vi "servo_motor_drive_computer.vi"() -> ()   [LabVIEW 2019]
uses:
  <vilib>/Platform/TimedLoop/XDataNode/timing_clust.ctl
  <vilib>/Platform/TimedLoop/XDataNode/nitl_modes.ctl
  <vilib>/Platform/TimedLoop/XDataNode/wakeup.ctl
  <vilib>/Utility/file.llb/Write Delimited Spreadsheet (DBL).vi
  <vilib>/Platform/TimedLoop/XDataNode/XDataNode.xnode
  <vilib>/myRIO/Common/Instrument Driver Framework/Utilities/typedefs/Generic FPGA Reference.ctl
  <vilib>/myRIO/Common/Instrument Driver Framework/Utilities/typedefs/myRIO v1.0 Reference.ctl
  <vilib>/myRIO/Common/Instrument Driver Framework/Utilities/typedefs/Hardware Version Enum.ctl
  <vilib>/myRIO/Common/Instrument Driver Framework/Utilities/typedefs/myRIO Generic Hardware Reference.ctl
  <vilib>/myRIO/Instrument Drivers/Onboard IO/PWM/PWM.lvlib
  <vilib>/myRIO/Instrument Drivers/Onboard IO/PWM/typedefs/PWM Configuration.ctl
  <vilib>/myRIO/Common/Instrument Driver Framework/myRIO v1.0/PWM/typedefs/PWM Channels Enum.ctl
  <vilib>/myRIO/Instrument Drivers/Onboard IO/PWM/typedefs/PWM Reference.ctl
  <vilib>/myRIO/Instrument Drivers/Onboard IO/PWM/vis/myRIO PWM Open.xnode
  <vilib>/myRIO/Instrument Drivers/Utilities/Utilities.lvlib
  <vilib>/myRIO/Common/Instrument Driver Framework/myRIO v1.0/PWM/vis/myRIO v1.1 Open PWM.vi
  <vilib>/userDefined/High Color/nirio_resource_hc.ctl
  <vilib>/myRIO/Express VI/Onboard IO/PWM/PWM Express VI.xnode
  <vilib>/myRIO/Common/Instrument Driver Framework/Utilities/vis/Is FPGA Ref Available.vi
  <vilib>/myRIO/Common/Instrument Driver Framework/myRIO v1.0/Encoder/typedefs/Encoder Count Direction Enum.ctl
  <vilib>/myRIO/Common/Instrument Driver Framework/myRIO v1.0/Encoder/typedefs/Encoder Signal Mode.ctl
  <vilib>/myRIO/Common/Instrument Driver Framework/myRIO v1.0/Encoder/typedefs/Encoder Channels Enum.ctl
  <vilib>/myRIO/Instrument Drivers/Onboard IO/Encoder/typedefs/Encoder Reference.ctl
  <vilib>/myRIO/Instrument Drivers/Onboard IO/Encoder/Encoder.lvlib
  <vilib>/myRIO/Instrument Drivers/Onboard IO/Encoder/vis/Read.vi
  <vilib>/myRIO/Common/Instrument Driver Framework/myRIO v1.0/Encoder/typedefs/Encoder Configuration v1.0.ctl
  <vilib>/myRIO/Common/Instrument Driver Framework/myRIO v1.0/Encoder/vis/myRIO v1.1 Open Encoder.vi
  <vilib>/myRIO/Common/Instrument Driver Framework/myRIO v1.0/Encoder/vis/myRIO v1.0 Configure Encoder.vi
  <vilib>/myRIO/Instrument Drivers/Onboard IO/Encoder/vis/myRIO Encoder Open.xnode
  <vilib>/myRIO/Express VI/Onboard IO/Encoder/Encoder Express VI.xnode
  <vilib>/Platform/TimedLoop/XDataNode/XDNodeRunTimeDep.lvlib
  <vilib>/myRIO/Common/Instrument Driver Framework/myRIO v1.0/DIO/typedefs/DIO Channels Enum.ctl
  <vilib>/myRIO/Common/Instrument Driver Framework/myRIO v1.0/DIO/typedefs/DIO Channels List.ctl
  <vilib>/myRIO/Instrument Drivers/Onboard IO/DIO/typedefs/DIO Reference.ctl
  <vilib>/myRIO/Instrument Drivers/Onboard IO/DIO/DIO.lvlib
  <vilib>/myRIO/Instrument Drivers/Onboard IO/DIO/vis/Write.vi
  <vilib>/myRIO/Common/Instrument Driver Framework/myRIO v1.0/DIO/vis/myRIO v1.1 Open DIO.vi
  <vilib>/myRIO/Instrument Drivers/Onboard IO/DIO/vis/myRIO DIO Open.xnode
  <vilib>/myRIO/Express VI/Onboard IO/DO/DO Express VI.xnode
panel:
  in  "file path (dialog if empty)":path
  in  "format (%.3f)":string="%.3f"
  out "velocity diff (deg/s)":dbl(graph)
  out "angle diff (deg)":dbl(graph)
  out "Duty cycle":dbl(graph)
  out "Time":dbl
  out "Angle_velocity(deg/s)":cluster{"set point":dbl, dbl}(graph)
  out "Angle_velocity(deg/s) Graph":dbl[][](graph)
  out "Angle(deg) Gragh":dbl[][](graph)
  out "Angle(deg)":cluster{dbl, dbl}(graph)
  out "Duty":dbl
  in  "stop":bool
  in  "Frequency [Hz]":dbl=1000.0
  in  "Gain 2":T1={"P Gain"=0.5, "I Gain"=0.0, "D Gain"=0.005}
  out "encoder_position":dbl
  out "Counter Value":i32
  in  "Encoder_Count":dbl=54991.0
  in  "t_shift":dbl=0.000125
  in  "T_ratio":dbl=1.0
  in  "buffer ratio":dbl=0.3
  in  "first or second tripod":bool
  in  "data of 5th order formula\nts,tair,a1-a6":dbl[](array[numeric])
  in  "Loop Period":i64=5
  out "duty cycle[%]":dbl
  out "pulse width[ms]":dbl
  in  "frequency":dbl=100.0
  out "offset":dbl
  in  "null offset":bool
  in  "position":dbl(slide) scale=-30.0..8.0
  in  "PWM channel":tag="A/PWM1"
  in  "stop":bool
  # "RC Servo Motor"
  # "v = 1; a = 15"
  # "v = 1.25; a = 15"
  # "v = 1.5; a = 15"
  # "0.184067181524967\n0.263820978418769\n256152.551336786\n-30272.30000274\n-9876.03760433421\n-1096.38594197941\n885.91817900106\n-44.6781799901984"
  # "0.215241998794118\n0.254514142390288\n4771.41078363533\n62185.8763006578\n-22508.5336527453\n390.805502041188\n686.695311017595\n-40.4128145310291"
  # "0.163616269216122\n0.27489641502463\n771965.39318528\n-201617.027694185\n8828.08396944145\n-2683.04589908678\n1085.57303422127\n-48.5860395324432"
  # "DC Motor"
  # "v = 1.75; a = 15"
  # "v = 2; a = 15"
  # "v = 2.25; a = 15"
  # "0.148651048423414\n0.288542414074344\n1776973.44893281\n-511591.467559457\n38775.9830765103\n-4576.94506688942\n1289.39828252671\n-52.3115561007577"
  # "0.136976185169818\n0.304016701267508\n3461279.85083822\n-993110.73746345\n80544.6579529191\n-6699.48295844177\n1494.82265451498\n-55.8934424469099"
  # "0.134381902205816\n0.369022171779704\n3272804.8365432\n-899365.569589567\n71225.2463409934\n-7039.10791102172\n1512.66147498591\n-59.3408899720725"
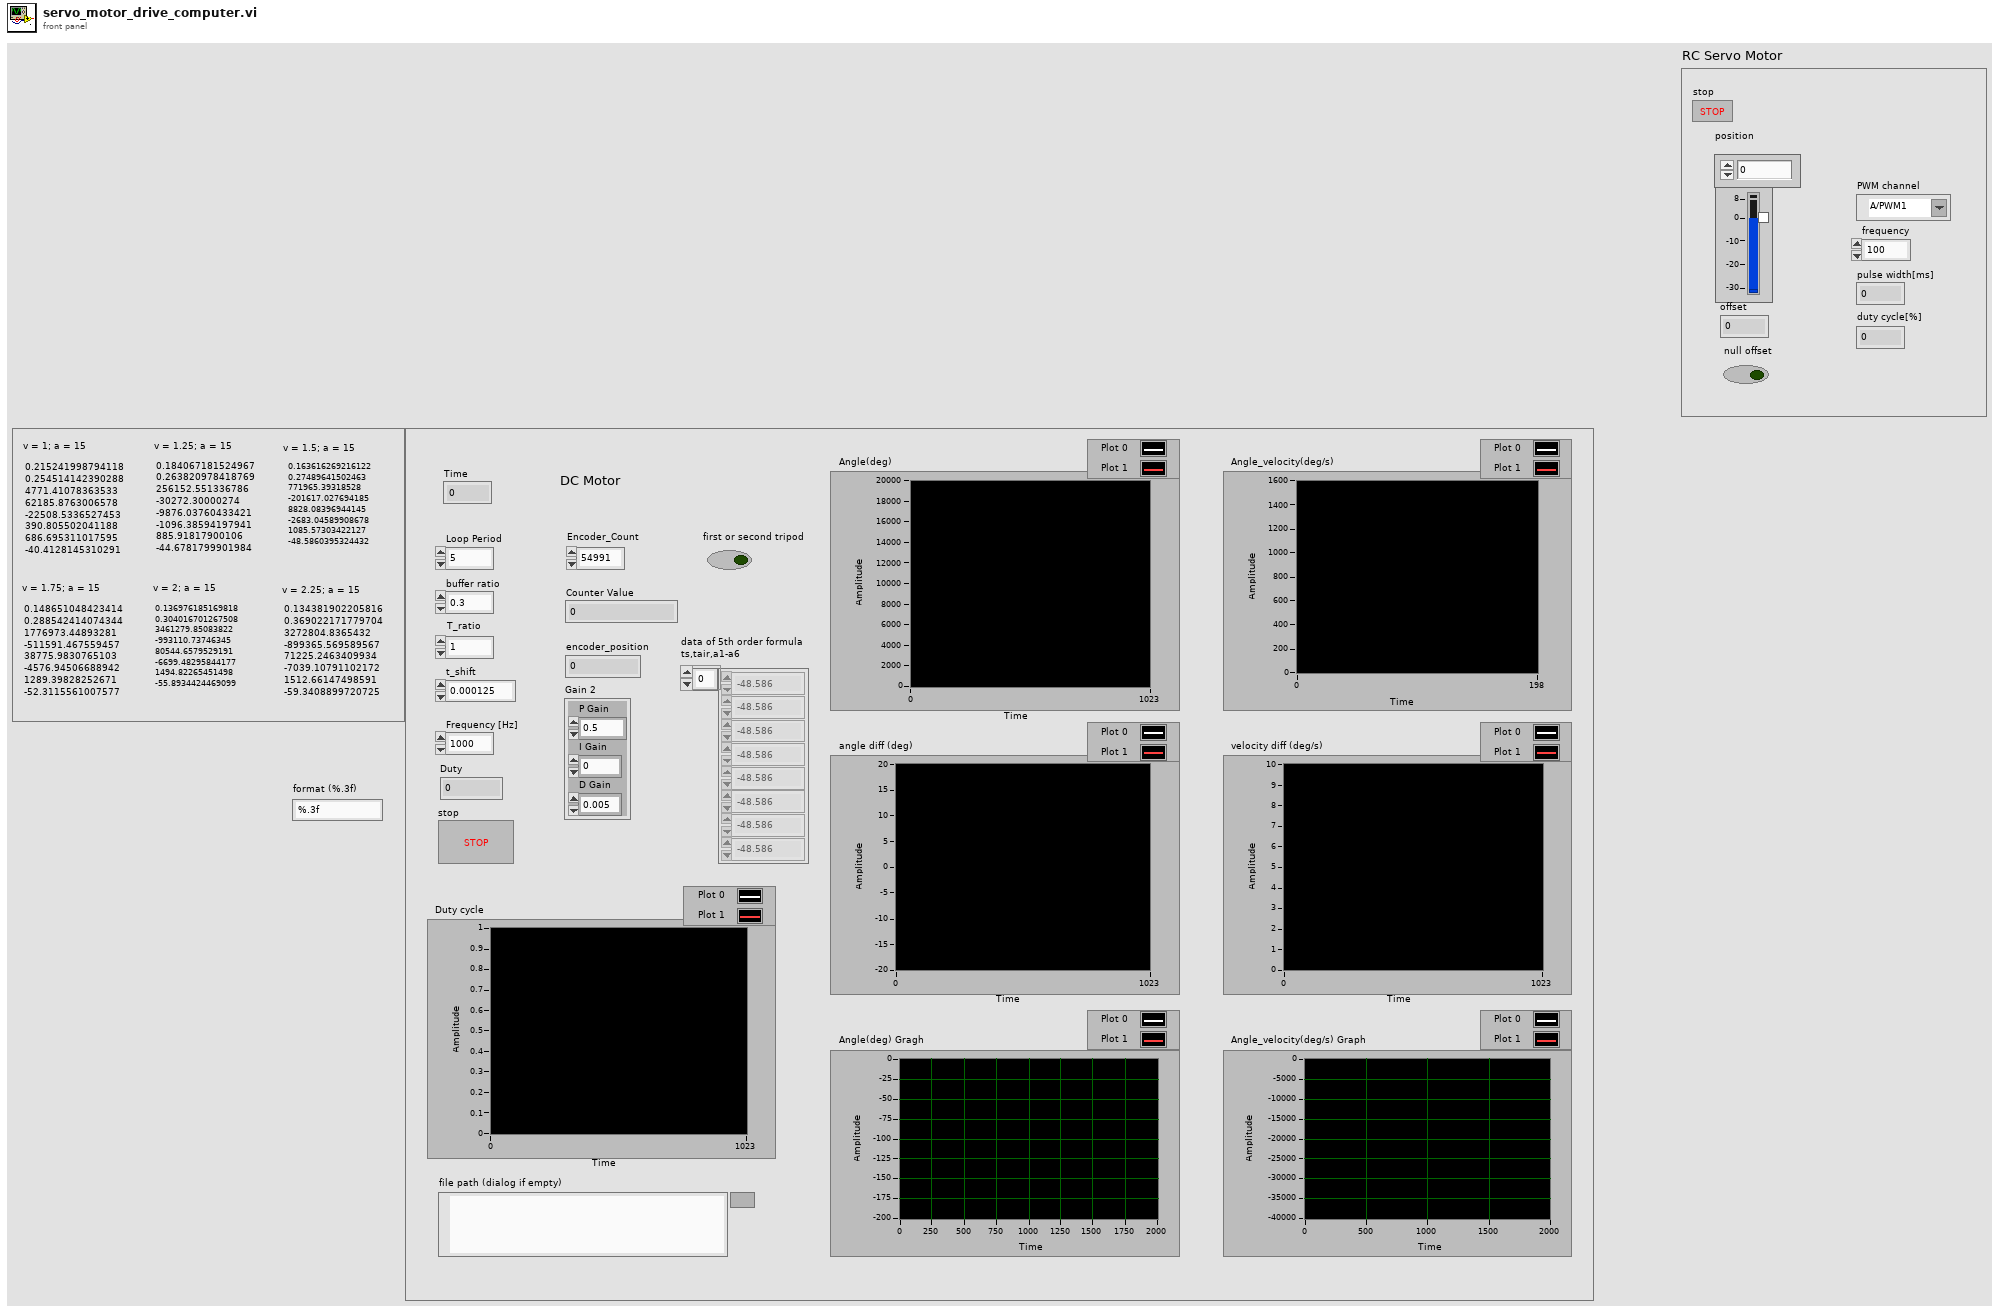
[diagram p1: front panel]
types:
  T1 = cluster{"P Gain":dbl, "I Gain":dbl, "D Gain":dbl}
  T2 = typedef "Encoder.lvlib/Encoder Reference.ctl" = cluster{"myRIO Reference":T3, "Encoder Channels Enum":T7}
  T3 = typedef "myRIO Generic Hardware Reference.ctl" = cluster{"myRIO Model":T4, "myRIO Hardware Reference":T5}
  T4 = typedef "Hardware Version Enum.ctl" = enum16{"Unknown", "myRIO-1900", "myRIO-1950", "roboRIO", "NI ELVIS RIO CM", "ELVIS III"}
  T5 = typedef "myRIO v1.0 Reference.ctl" = cluster{"Generic FPGA Reference":T6, "Allow multiple opens":bool}
  T6 = typedef "Generic FPGA Reference.ctl" = refnum<k20>
  T7 = typedef "Encoder Channels Enum.ctl" = enum16{"Not Connected", "C/ENC0", "C/ENC1", "A/ENC", "A/ENC0", "A/ENC1", "A/ENC2", "A/ENC3", "A/ENC4", "A/ENC5", "A/ENC6", "A/ENC7", "A/ENC8", "A/ENC9", "B/ENC", "B/ENC0", "B/ENC1", "B/ENC2", "B/ENC3", "B/ENC4", "B/ENC5", "B/ENC6", "B/ENC7", "B/ENC8", "B/ENC9", "DIO/ENC0", "DIO/ENC1", "DIO/ENC2", "DIO/ENC3", "DIO/ENC4"}
  T8 = typedef "Encoder Signal Mode.ctl" = enum16{"Quadrature phase signal", "Step and direction signal"}
  T9 = typedef "nirio_resource_hc.ctl" = tag
  T10 = cluster{"set position":dbl, "set position":dbl, "set position":dbl, "set position":dbl, "set position":dbl, "set position":dbl}
  T11 = typedef "PWM.lvlib/PWM Reference.ctl" = cluster{"myRIO Reference":T3, "PWM Channels Enum":T12, "PWM Configuration":T13}
  T12 = typedef "PWM Channels Enum.ctl" = enum16{"Not Connected", "C/PWM0", "C/PWM1", "A/PWM0", "A/PWM1", "A/PWM2", "A/PWM3", "A/PWM4", "A/PWM5", "A/PWM6", "A/PWM7", "A/PWM8", "A/PWM9", "A/PWM10", "A/PWM11", "A/PWM12", "A/PWM13", "A/PWM14", "A/PWM15", "A/PWM16", "A/PWM17", "A/PWM18", "A/PWM19", "B/PWM0", "B/PWM1", "B/PWM2", "B/PWM3", "B/PWM4", "B/PWM5", "B/PWM6", "B/PWM7", "B/PWM8", "B/PWM9", "B/PWM10", "B/PWM11", "B/PWM12", "B/PWM13", "B/PWM14", "B/PWM15", "B/PWM16", "B/PWM17", "B/PWM18", "B/PWM19", "PWM/PWM0", "PWM/PWM1", "PWM/PWM2", "PWM/PWM3", "PWM/PWM4", "PWM/PWM5", "PWM/PWM6", "PWM/PWM7", "PWM/PWM8", "PWM/PWM9"}
  T13 = typedef "PWM.lvlib/PWM Configuration.ctl" = cluster{"Frequency":dbl, "Duty Cycle":dbl}
  T14 = typedef "DIO.lvlib/DIO Reference.ctl" = cluster{"myRIO Reference":T3, "DIO Channels List":T15}
  T15 = typedef "DIO Channels List.ctl" = T16[]
  T16 = typedef "DIO Channels Enum.ctl" = enum16{"Not Connected", "C/DIO0", "C/DIO1", "C/DIO2", "C/DIO3", "C/DIO4", "C/DIO5", "C/DIO6", "C/DIO7", "A/DIO0", "A/DIO1", "A/DIO2", "A/DIO3", "A/DIO4", "A/DIO5", "A/DIO6", "A/DIO7", "A/DIO8", "A/DIO9", "A/DIO10", "A/DIO11", "A/DIO12", "A/DIO13", "A/DIO14", "A/DIO15", "A/DIO16", "A/DIO17", "A/DIO18", "A/DIO19", "B/DIO0", "B/DIO1", "B/DIO2", "B/DIO3", "B/DIO4", "B/DIO5", "B/DIO6", "B/DIO7", "B/DIO8", "B/DIO9", "B/DIO10", "B/DIO11", "B/DIO12", "B/DIO13", "B/DIO14", "B/DIO15", "B/DIO16", "B/DIO17", "B/DIO18", "B/DIO19", "LED0", "LED1", "LED2", "LED3", "Button0", "DIO/DIO0", "DIO/DIO1", "DIO/DIO2", "DIO/DIO3", "DIO/DIO4", "DIO/DIO5", "DIO/DIO6", "DIO/DIO7", "DIO/DIO8", "DIO/DIO9", "SPI/CS0", "SPI/CS1", "SPI/CS2", "SPI/CS3", "LED RADIO (Green)", "LED RADIO (Red)", "LED COMM (Green)", "LED COMM (Red)", "LED MODE (Green)", "LED MODE (Red)"}
  T17 = typedef "XDNodeRunTimeDep.lvlib/timing_clust.ctl" = cluster{"Expected End [f-1]":u64, "Actual End [f-1]":u64, "Finished Late? [f-1]":bool, "Expected End [i-1]":u64, "Actual End [i-1]":u64, "Finished Late? [i-1]":bool, "Expected Start [i]":u64, "Actual Start [i]":u64, "Expected Start [f]":u64, "Actual Start [f]":u64, "Source Name":string, "Structure Name":string, "Period":i64, "Deadline":i64, "Offset":i64, "Start":i64, "Priority":i32, "Timeout":i32, "Mode":T18, "Wakeup Reason":T19, "Error":errorcluster, "Source Type":string, "Secondary Source Type":string, "Global End Time":u64, "Global Start Time":u64, "Frame Duration":u64, "Iteration Duration":u64, "Assigned CPU":i32, "I/O Scan Engine Mode":u32}
  T18 = typedef "XDNodeRunTimeDep.lvlib/nitl_modes.ctl" = enum32{"No Change", "Process missed periods, maintain original phase", "Discard missed periods, maintain original phase", "Process missed periods, ignore original phase", "Discard missed periods, ignore original phase"}
  T19 = typedef "XDNodeRunTimeDep.lvlib/wakeup.ctl" = enum32{"Normal", "Aborted", "Asynchronous wakeup", "Timing source error", "Timed loop error", "Timeout"}
  T20 = cluster{"[0]":dbl, "[1]":dbl, "[2]":dbl, "[3]":dbl, "[4]":dbl, "[5]":dbl}
  T21 = cluster{"set position":i32, "set position":i32, "set position":i32, "set position":i32, "set position":i32, "set position":i32}
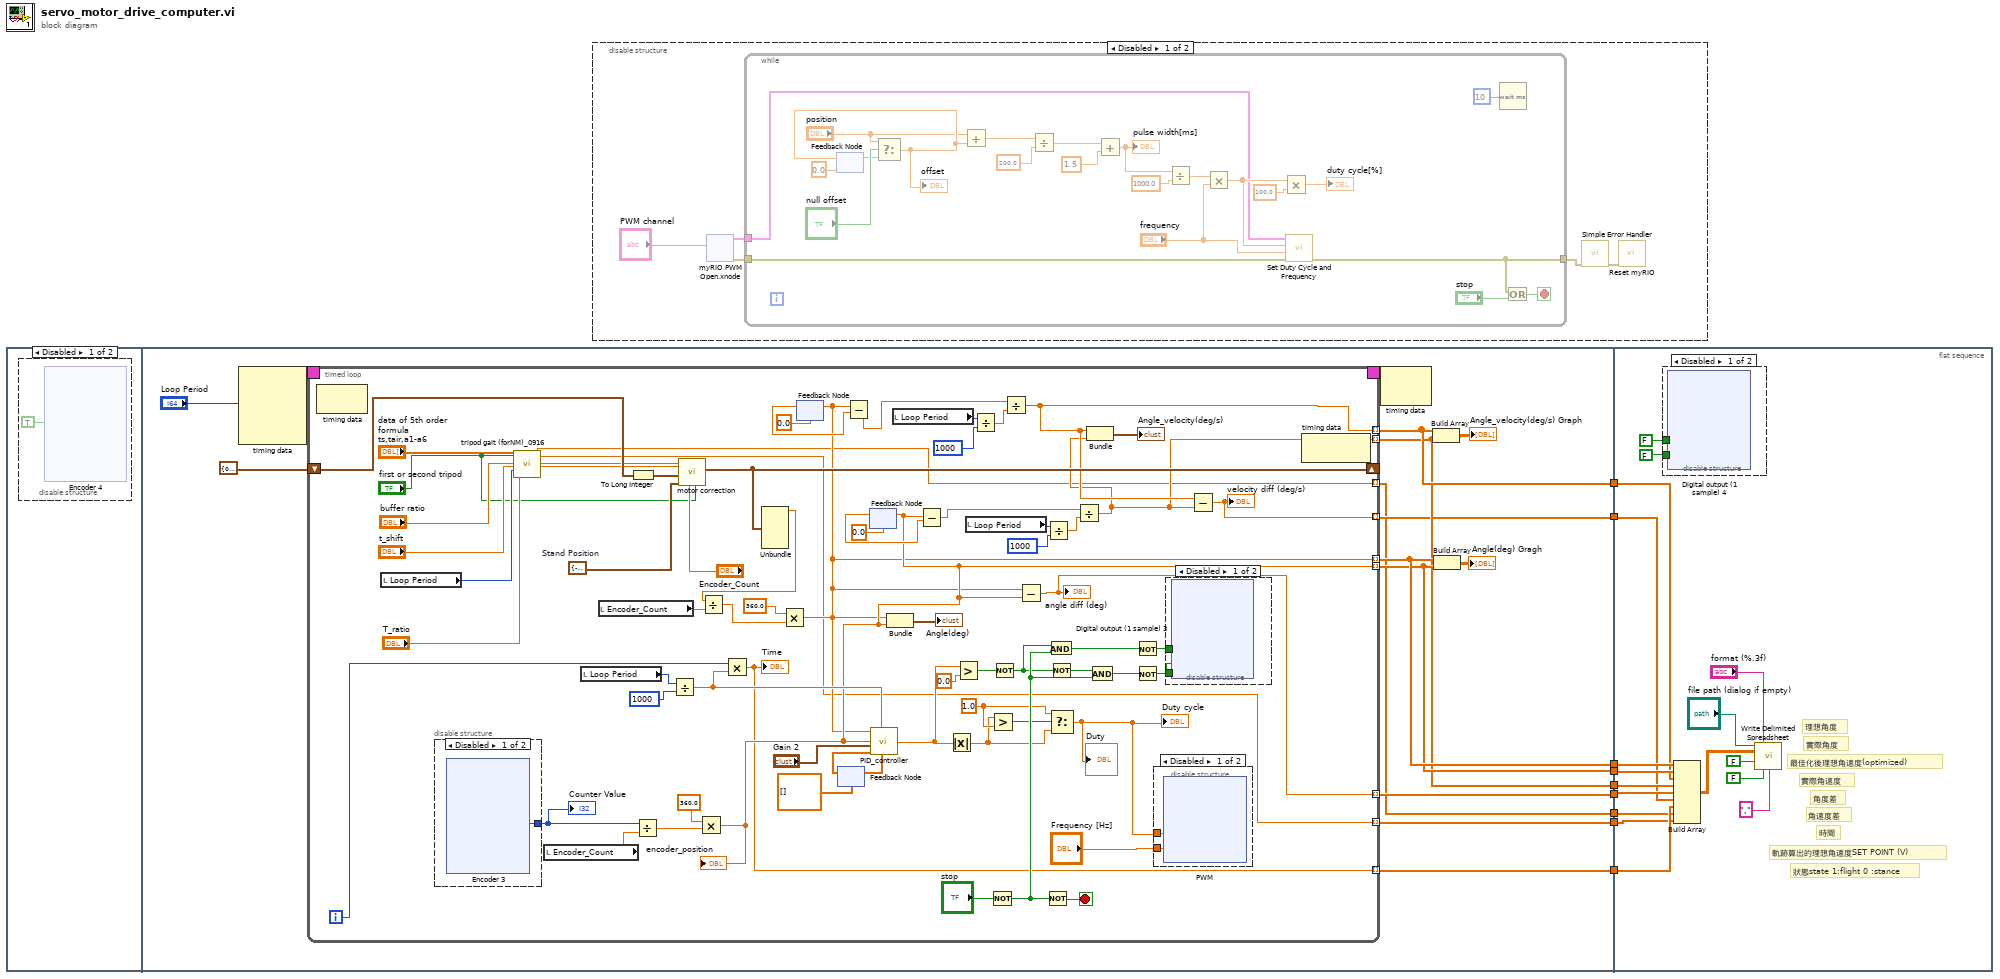
[diagram p0: block diagram]
diagram:
  n1 = flat-sequence {
    tunnel: [w65] -> w9
    tunnel: [w64] -> w8
    tunnel: [w63] -> w7
    tunnel: [w62] -> w6
    tunnel: [w61] -> w5
    tunnel: [w60] -> w4
    tunnel: [w59] -> w3
    tunnel: [w58] -> w2
    tunnel: [w57] -> w1
    tunnel: w9 -> [w282]
    tunnel: w8 -> [w281]
    tunnel: w7 -> [w280]
    tunnel: w6 -> [w279]
    tunnel: w5 -> [w278]
    tunnel: w4 -> [w277]
    tunnel: w3 -> [w275]
    tunnel: w2 -> [w270]
    tunnel: w1 -> [w269]
    frame #0 {
      n2 = disable-structure shown="Disabled" {
        frame Disabled {
          n3 = xnode "Encoder 4"("Reset Counter"=TRUE) -> ()  [unwired: 1 in, 4 out]
        }
        frame Enabled {
        }
      }
    }
    frame #1 {
      n4 = node-c288("Loop Period") -> (w71:T17)  [unwired: 3 in]
      n5 = timed-loop {
        timing: w71 -> [_]
        timing-out: [_] -> w70
        shift-right: [w132] -> _
        shift-left: T10 {"set position"=0.0, "set position"=0.0, "set position"=0.0, "set position"=0.0, "set position"=0.0, "set position"=0.0} ("Setpoint_to_motor") -> [w130]
        tunnel: [w82] -> w64 mode=indexing
        tunnel: [w79] -> w65 mode=indexing
        tunnel: [w80] -> w62 mode=indexing
        tunnel: [w81] -> w63 mode=indexing
        tunnel: [w78] -> w61 mode=indexing
        tunnel: [w77] -> w60 mode=indexing
        tunnel: [w76] -> w59 mode=indexing
        tunnel: [w75] -> w58 mode=indexing
        tunnel: [w74] -> w57 mode=indexing
        i -> [w89]
        stop <- w109 stop-if-true
        w117 = 1.0 ("y")
        w129 = T20 {"[0]"=-27495.5, "[1]"=-27495.5, "[2]"=-27495.5, "[3]"=-27495.5, "[4]"=-27495.5, "[5]"=-27495.5}  # Stand Position
        n6 = node-c288() -> ()  [unwired: 1 in, 1 out]
        n7 = local read "Loop Period"() -> (w136:i64)
        n8 = disable-structure shown="Disabled" {
          disable-tunnel: [w216 _] -> w84
          frame Disabled {
            n9 = xnode "Encoder 3"() -> ("Counter Value"=w216:i32)  [unwired: 2 in, 3 out]
          }
          frame Enabled {
          }
        }
        "Counter Value" <- w84
        n10 = call "tripod gait (forNM)_0916.vi"("data of 5th order formula\nts,tair,a1-a6"="data of 5th order formula\nts,tair,a1-a6", "first or second"="first or second tripod", "buffer ratio"="buffer ratio", "t_shift"="t_shift", "sample time"=w136, "T_ratio"="T_ratio") -> ("SET POINT V"=w75:dbl, "state 2"=w74:dbl, "Set Point"=w73:dbl, "Set Point 2"=w92:dbl)  [unwired: 4 in, 14 out]
        n11 = local read "Encoder_Count"() -> (w133:dbl)
        n12 = local read "Loop Period"() -> (w100:i64)
        n13 = local read "Encoder_Count"() -> (w98:dbl)
        n14 = To Long Integer(number=w130) -> (32bit integer=w131:T21)
        n15 = Divide(x=w84, y=w133) -> (x/y=w93:dbl)
        n16 = Divide(x=w100, y=i64 1000) -> (x/y=w90:dbl)
        n17 = call "motor correction.vi"("first or second"="first or second tripod", "Encoder_Count"="Encoder_Count", "Stand Position"=w129, "encoder position"=w131, "set position 2"=w92, "set position"=w73) -> ("Setpoint_to_motor"=w132:T10)  [unwired: 4 in, 1 out]
        n18 = Multiply(x=360.0, y=w93) -> (x*y=w82:dbl)
        "encoder_position" <- w82
        n19 = Multiply(x=w89, y=w90) -> (x*y=w76:dbl)
        "Time" <- w76
        n20 = Unbundle(w132) -> ("set position"=w72:dbl)  [unwired: 5 out]
        n21 = Divide(x=w72, y=w98) -> (x/y=w96:dbl)
        n22 = Multiply(x=360.0, y=w96) -> (x*y=w79:dbl)
        n23 = feedback #1(0.0) -> (w104:dbl)
        n24 = feedback-in #1(w79) -> ()
        n25 = feedback #2(dbl[] [] ("state(k)")) -> (w128:dbl[])
        n26 = Subtract(x=w79, y=w104) -> (x-y=w87:dbl)
        n27 = feedback #3(0.0) -> (w86:dbl)
        n28 = feedback-in #3(w82) -> ()
        n29 = call "PID_controller.vi"("Time Period"=w90, "state(k-1)"=w128, "Gain"="Gain 2", "variable"=w82, "set point"=w79) -> ("PID gain"=w110:dbl, "state(k)"=w127:dbl[])
        n30 = feedback-in #2(w127) -> ()
        n31 = Bundle(w79, w82) -> (→"Angle(deg)":cluster{dbl, dbl})  [unwired: 1 in]
        n32 = local read "Loop Period"() -> (w103:i64)
        n33 = Subtract(x=w82, y=w86) -> (x-y=w88:dbl)
        n34 = Absolute Value(x=w110) -> (abs(x)=w116:dbl)
        n35 = Greater?(x=w110, y=0.0) -> (0:w119:bool)
        n36 = local read "Loop Period"() -> (w107:i64)
        n37 = Divide(x=w103, y=i64 1000) -> (x/y=w102:dbl)
        n38 = Not(x="stop") -> (.not. x?=w121:bool)
        n39 = Greater?(x=w116, y=w117) -> (0:w118:bool)
        n40 = Not(x=w119) -> (.not. x?=w115:bool)
        n41 = Divide(x=w87, y=w102) -> (x/y=w81:dbl)
        n42 = Subtract(x=w79, y=w82) -> (x-y=w78:dbl)
        "angle diff (deg)" <- w78
        n43 = Not(x=w121) -> (.not. x?=w109:bool)
        n44 = Divide(x=w107, y=i64 1000) -> (x/y=w105:dbl)
        n45 = And(x=w115, y=w121) -> (x .and. y?=w112:bool)
        n46 = Not(x=w115) -> (.not. x?=w123:bool)
        n47 = Select(t=w117, s=w118, f=w116) -> (s? t:f=w83:dbl)
        "Duty" <- w83
        "Duty cycle" <- w83
        n48 = Divide(x=w88, y=w105) -> (x/y=w80:dbl)
        n49 = Bundle(w81, w80) -> (→"Angle_velocity(deg/s)":cluster{dbl, dbl})  [unwired: 1 in]
        n50 = And(x=w123, y=w121) -> (x .and. y?=w114:bool)
        n51 = Not(x=w112) -> (.not. x?=w111:bool)
        n52 = Not(x=w114) -> (.not. x?=w113:bool)
        n53 = disable-structure shown="Disabled" {
          disable-tunnel: "Frequency [Hz]" -> [w142 _]
          disable-tunnel: w83 -> [w141 _]
          frame Disabled {
            n54 = xnode "PWM"("Duty Cycle"=w141, "Frequency [Hz]"=w142) -> ()  [unwired: 1 in, 1 out]
          }
          frame Enabled {
          }
        }
        n55 = disable-structure shown="Disabled" {
          disable-tunnel: w113 -> [w179 _]
          disable-tunnel: w111 -> [w178 _]
          frame Disabled {
            n56 = xnode "Digital output (1 sample) 3"("A/DIO0 (Pin 11)"=w178, "A/DIO1 (Pin 13)"=w179) -> ()  [unwired: 1 in, 1 out]
          }
          frame Enabled {
          }
        }
        n57 = Subtract(x=w81, y=w80) -> (x-y=w77:dbl)
        "velocity diff (deg/s)" <- w77
        n58 = node-c288() -> ()  [unwired: 1 in, 1 out]
      }
      n59 = node-c288(w70) -> ()  [unwired: 1 out]
      n60 = Build Array(w63, w62) -> (→"Angle_velocity(deg/s) Graph":dbl[][])
      n61 = Build Array(w65, w64) -> (→"Angle(deg) Gragh":dbl[][])
    }
    frame #2 {
      # "狀態state 1:flight 0 :stance"
      # "軌跡算出的理想角速度SET POINT (V)"
      # "時間"
      # "角速度差"
      # "角度差"
      # "實際角度"
      # "理想角度"
      # "實際角速度"
      # "最佳化後理想角速度(optimized)"
      n62 = disable-structure shown="Disabled" {
        disable-tunnel: FALSE ("A/DIO0 (Pin 11)") -> [w287 _]
        disable-tunnel: FALSE ("A/DIO1 (Pin 13)") -> [w286 _]
        frame Disabled {
          n63 = xnode "Digital output (1 sample) 4"("A/DIO0 (Pin 11)"=w287, "A/DIO1 (Pin 13)"=w286) -> ()  [unwired: 1 in, 1 out]
        }
        frame Enabled {
        }
      }
      n64 = Build Array(w282, w281, w280, w279, w278, w277, w275, w270, w269) -> (w276:dbl[][])
      n65 = call-poly <vilib>:"Write Delimited Spreadsheet.vi"("file path (dialog if empty)"="file path (dialog if empty)", "format (%.3f)"="format (%.3f)", "2D data"=w276, "append to file? (new file:F)"=FALSE, "transpose? (no:F)"=FALSE, "delimiter (\\t)"="," ("delimiter (\\t)")) -> ()  [unwired: 8 in, 2 out]
    }
  }
  n66 = disable-structure shown="Disabled" {
    frame Disabled {
      n67 = xnode "myRIO PWM Open.xnode"("Channel Name"="PWM channel") -> ("error out"=w326:errorcluster, "PWM Ref Out"=w327:T11)  [unwired: 2 in]
      n68 = while {
        tunnel: w327 -> [w351]
        tunnel: w326 -> [w350]
        tunnel: [w349] -> w325
        stop <- w347 stop-if-true
        n69 = feedback #4(0.0 ("Numeric")) -> (w364:dbl)
        n70 = Select(t="position", s="null offset", f=w364) -> (s? t:f=w363:dbl)
        "offset" <- w363
        n71 = feedback-in #4(w363) -> ()
        n72 = Add(x="position", y=w363) -> (x+y=w362:dbl)
        n73 = Divide(x=w362, y=200.0) -> (x/y=w360:dbl)
        n74 = Add(x=w360, y=1.5) -> (x+y=w358:dbl)
        "pulse width[ms]" <- w358
        n75 = Divide(x=w358, y=1000.0) -> (x/y=w356:dbl)
        n76 = Multiply(x=w356, y="frequency") -> (x*y=w354:dbl)
        n77 = Multiply(x=w354, y=100.0) -> (x*y=→"duty cycle[%]":dbl)
        n78 = call <vilib>:"Set Duty Cycle and Frequency.vi"("error in (no error)"=w350, "Frequency [Hz]"="frequency", "Duty Cycle"=w354, "PWM Ref In"=w351) -> ("error out"=w349:errorcluster)  [unwired: 5 in, 1 out]
        n79 = Wait (ms)(milliseconds to wait=u32 10) -> ()  [unwired: 1 out]
        n80 = Or(x=w349, y="stop") -> (x .or. y?=w347:bool)
      }
      n81 = call <vilib>:"Simple Error Handler.vi"("error in (no error)"=w325) -> ("error out"=w324:errorcluster)  [unwired: 4 in, 4 out]
      n82 = call <vilib>:"Reset myRIO.vi"("error in (no error)"=w324) -> ()  [unwired: 10 in, 1 out]
    }
    frame Enabled {
    }
  }
